vi "LEBITplc.UpdateMonDep.vi"(0 "i ref in":refnum<vi>, 1 "data":dbl, 2 "i attribute":T1, 3 "DependentMonitors":string[](array[string]), 5 "error in":errorcluster, 6 "quality":i32, 9 "no link":bool) -> (14 "i ref out":refnum<vi>, 16 "i attribute out":T1, 19 "error out":errorcluster)   [LabVIEW 2014, in "LEBITplc.lvlib"]
uses:
  LEBITplc.lvlib
  LEBITplc.i attribute.ctl
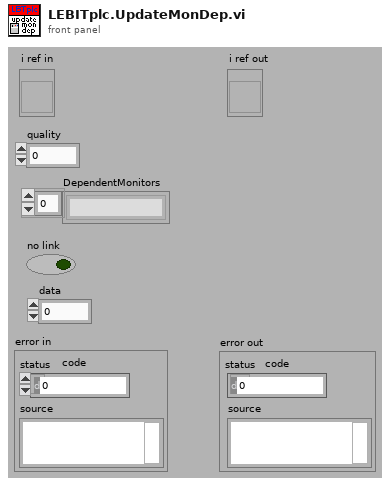
[diagram p1: front panel]
types:
  T1 = typedef "LEBITplc.lvlib/LEBITplc.i attribute.ctl" = cluster{"LLFLocation":string, "SetFileLocation":string, "nickNames":string[], "setValuePLCServiceID":i32[], "GUIServiceID":i32[], "monValuePLC":string[], "SetValueServiceID":i32[], "MonValueServiceID":i32[], "SetValue":dbl[][], "SetValueMin":dbl[], "SetValueMax":dbl[], "SetValueInfoServiceID":i32[], "GUINames":string[], "ListOfBases":string[], "Scale":dbl[], "Offset":dbl[], "setValuePLC":string[], "BaseName":string[], "ScaleServiceID":i32[], "OffsetServiceID":i32[], "AllPLCValues":string[], "CondSpecialArray":string[][], "CondSpecialIndex":i32[], "CondSpecialMonValue":dbl[], "RecentlyChanged":i32[], "SetFileLocationID":i32, "Dependent-Monitors":string[][], "LastLoadedFiles":string[], "IonGuideCalibLocation":string, "Monitor Dependent":string[], "Special":string[], "PLC?":bool[], "Start Date":string, "ListOfBasesServiceID":i32, "SETRA VISA resource":refnum<visa-resource-name>}
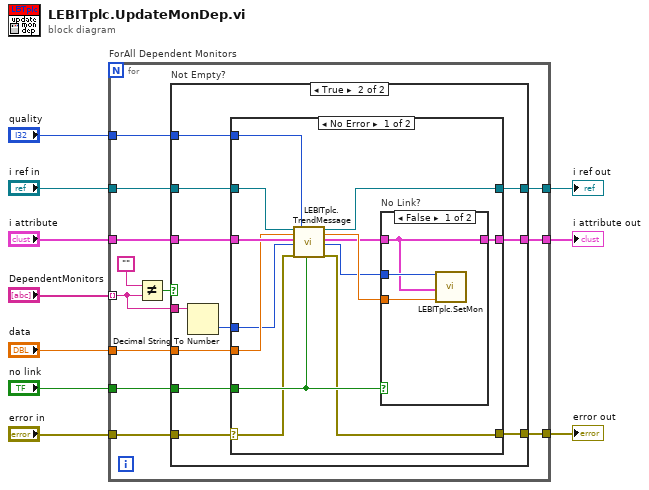
[diagram p0: block diagram]
diagram:
  n1 = for "ForAll Dependent Monitors" {
    tunnel: "no link" -> [w22]
    tunnel: [w21] -> w9
    tunnel: "i attribute" -> [w20]
    tunnel: "error in" -> [w19]
    tunnel: "i ref in" -> [w18]
    tunnel: [w17] -> w5
    tunnel: "DependentMonitors" -> [w11] mode=indexing
    tunnel: [w16] -> w4
    tunnel: "data" -> [w15]
    tunnel: "quality" -> [w14]
    n2 = Not Equal?(x="", y=w11) -> (x != y?=w12:bool)
    n3 = case "Not Empty?" shown="True" w12 {
      tunnel: w22 -> [_ w36]
      tunnel: [w23 w35] -> w21
      tunnel: w20 -> [w24 w34]
      tunnel: w19 -> [w23 w33]
      tunnel: w18 -> [w25 w32]
      tunnel: [w25 w31] -> w17
      tunnel: [w24 w30] -> w16
      tunnel: w15 -> [_ w29]
      tunnel: w14 -> [_ w28]
      tunnel: w11 -> [_ w26]
      frame False {
      }
      frame True {
        n4 = Decimal String To Number(string=w26) -> (number=w27:i32)  [unwired: 2 in, 1 out]
        n5 = case shown="No Error" w33 {
          selector: w33 -> [w40 w55]
          tunnel: w36 -> [w43 _]
          tunnel: [w39 w55] -> w35
          tunnel: w29 -> [w46 _]
          tunnel: w34 -> [w47 w53]
          tunnel: w32 -> [w45 w54]
          tunnel: [w44 w54] -> w31
          tunnel: [w48 w53] -> w30
          tunnel: w28 -> [w38 _]
          tunnel: w27 -> [w37 _]
          frame No Error {
            n6 = call "LEBITplc.TrendMessage.vi"("i ref in"=w45, "data"=w46, "i attribute"=w47, "index"=w37, "error in"=w40, "quality"=w38, "no link"=w43) -> ("i ref out"=w44:refnum<vi>, "data out"=w42:dbl, "i attribute out"=w41:T1, "error out"=w39:errorcluster)  [unwired: 9 in]
            n7 = case "No Link?" shown="False" w43 {
              tunnel: w42 -> [w51 _]
              tunnel: w41 -> [w49 w52]
              tunnel: [w49 w52] -> w48
              tunnel: w37 -> [w50 _]
              frame False {
                n8 = call "LEBITplc.SetMon.vi"("index of element"=w50, "i attribute in"=w49, "Data"=w51) -> ()  [unwired: 17 in]
              }
              frame True {
              }
            }
          }
          frame Error {
          }
        }
      }
    }
  }
  "error out" <- w9
  "i ref out" <- w5
  "i attribute out" <- w4
